vi "CAENHV Get Bd Param Bitfield.vi"(8 "error in (no error)":errorcluster, 9 "ParName":string, 10 "slot":u16, 11 "handle":i32) -> (0 "error out":errorcluster, 3 "ParVal":bool[](array[boolean]))   [LabVIEW 2009, in "CAENHVWrapper.lvlib"]
doc: "CAENHVLIB_API CAENHVRESULT CAENHV_GetBdParam(int handle, \n ushort slotNum, const ushort *slotList, const char *ParName, void *ParValList);"
uses:
  <userlib>/CAENHVWrapper/CAENHVWrapper.lvlib
  <userlib>/CAENHVWrapper/CAENHVWrapper.dll
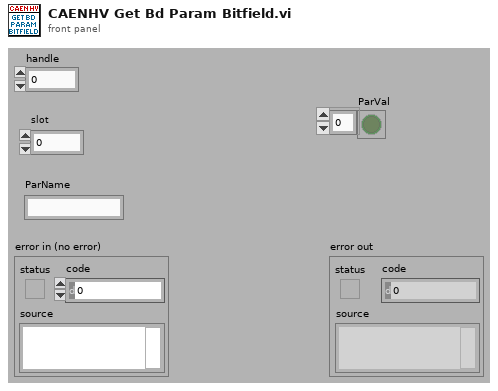
[diagram p1: front panel]
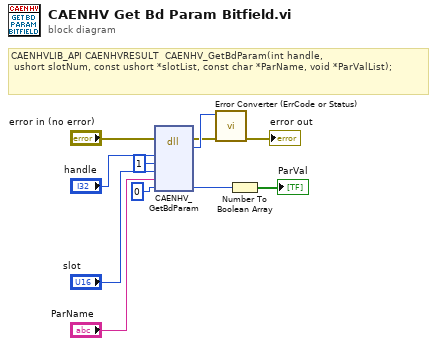
[diagram p0: block diagram]
diagram:
  # "CAENHVLIB_API CAENHVRESULT  CAENHV_GetBdParam(int handle, \n ushort slotNum, const ushort *slotList, const char *ParName, void *ParValList);"
  n1 = dll-call lib="C:/Program Files/National Instruments/LabVIEW 2009/user.lib/CAENHVWrapper/CAENHVWrapper.*" fn="CAENHV_GetBdParam"(error in="error in (no error)", "handle"="handle", "slotNum"=u16 1, "slotList"="slot", "ParName"="ParName", "ParValList"=u32 0) -> (error out=w5:errorcluster, "return type"=w6:i32, "ParValList"=w3:u32)  [unwired: 6 in, 1 out]
  n2 = call <userlib>:"Error Converter (ErrCode or Status).vi"("error in (no error)"=w5, "error code"=w6) -> ("error out"=→"error out":errorcluster)  [unwired: 9 in]
  n3 = Number To Boolean Array(number=w3) -> (Boolean array=→"ParVal":bool[])
